vi "Initialize VDI synthesizers.vi"(11 "VDI config constants in":T3[](array[typedef])) -> (2 "Status":T1, 3 "VDI config constants out":T3[](array[typedef]))   [LabVIEW 2024, in "THz source modeule.lvlib"]
uses:
  THz source modeule.lvlib
  ctl/THz MW generator constants.ctl
  ctl/VDI status.ctl
  ctl/Synth status.ctl
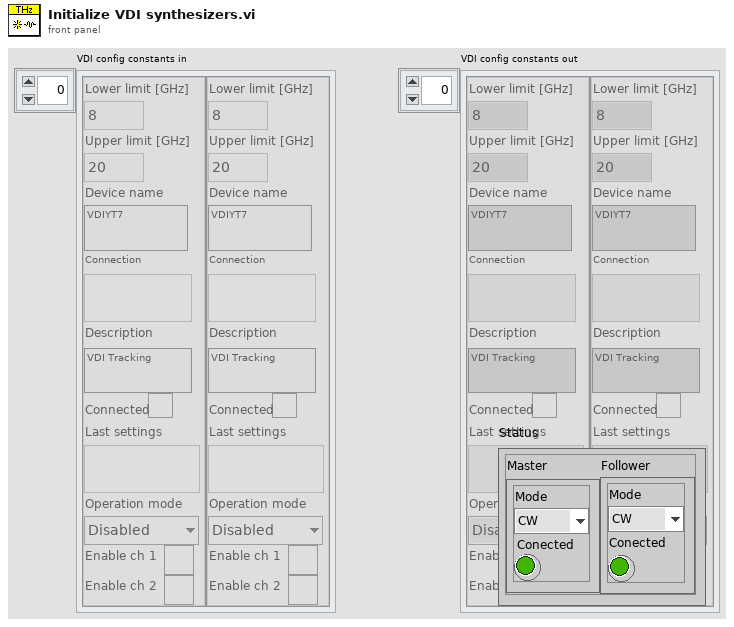
[diagram p1: front panel]
types:
  T1 = typedef "THz source modeule.lvlib/VDI status.ctl" = cluster{"Master":T2, "Follower":T2}
  T2 = typedef "THz source modeule.lvlib/Synth status.ctl" = cluster{"Mode":enum16{"CW", "Sweep"}, "Conected":bool}
  T3 = typedef "THz source modeule.lvlib/THz MW generator constants.ctl" = cluster{"Lower limit [GHz]":dbl, "Upper limit [GHz]":dbl, "Device name":string, "Connection":string, "Description":string, "Connected":bool, "Last settings":string, "Operation mode":enum16{"Disabled", "CW", "Arbitrary", "Sweep"}, "Enable ch 1":bool, "Enable ch 2":bool}
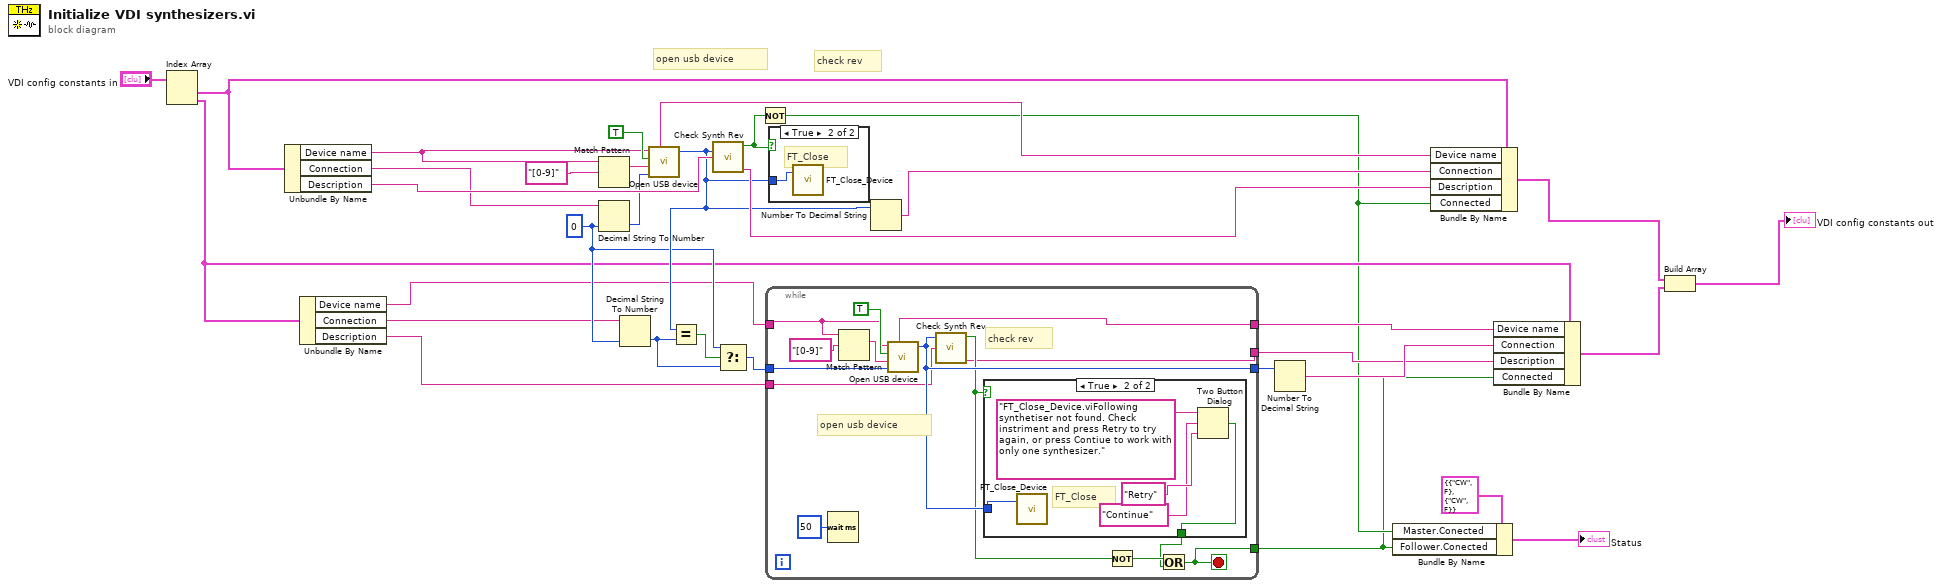
[diagram p0: block diagram]
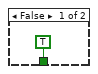
[diagram p2: hidden frame]
diagram:
  w15 = u64 0 ("default (0 I32)")
  # "check rev"
  # "open usb device"
  n1 = Index Array(array="VDI config constants in") -> (element #1=w14:T3, element #2=w7:T3)  [unwired: 2 in]
  n2 = Unbundle By Name(w14) -> ("Device name"=w6:string, "Connection"=w19:string, "Description"=w26:string)
  n3 = Unbundle By Name(w7) -> ("Device name"=w11:string, "Connection"=w12:string, "Description"=w13:string)
  n4 = Match Pattern(string=w6, regular expression="[0-9]") -> (match substring=w28:string)  [unwired: 1 in, 3 out]
  n5 = Decimal String To Number(string=w19, default (0L)=w15) -> (number=w18:u64)  [unwired: 1 in, 1 out]
  n6 = Decimal String To Number(string=w12, default (0L)=w15) -> (number=w16:u64)  [unwired: 1 in, 1 out]
  n7 = call <instrlib>:"Open USB device.vi"("SN#"=w6, "close first"=TRUE, "Prefix"=w28, "Old handle"=w18) -> ("SN# out"=w27:string, "Handle out"=w20:u64)  [unwired: 2 out]
  n8 = Equal?(x=w20, y=w16) -> (x = y?=w23:bool)
  n9 = call <instrlib>:"Check Synth Rev.vi"("Handle"=w20, "Description"=w26) -> ("Wrong Rev"=w21:bool, "Device Description"=w24:string)  [unwired: 7 in]
  n10 = Select(t=w15, s=w23, f=w16) -> (s? t:f=w22:u64)
  n11 = Not(x=w21) -> (.not. x?=w2:bool)
  n12 = while {
    tunnel: [w45] -> w1
    tunnel: w11 -> [w41]
    tunnel: [w38] -> w10
    tunnel: w13 -> [w35]
    tunnel: [w34] -> w8
    tunnel: w22 -> [w39]
    tunnel: [w37] -> w32
    stop <- w45 stop-if-true
    # "check rev"
    # "open usb device"
    n13 = Wait (ms)(milliseconds to wait=u32 50) -> ()  [unwired: 1 out]
    n14 = Match Pattern(string=w41, regular expression="[0-9]") -> (match substring=w40:string)  [unwired: 1 in, 3 out]
    n15 = call <instrlib>:"Open USB device.vi"("SN#"=w41, "close first"=TRUE, "Prefix"=w40, "Old handle"=w39) -> ("SN# out"=w38:string, "Handle out"=w37:u64)  [unwired: 2 out]
    n16 = call <instrlib>:"Check Synth Rev.vi"("Handle"=w37, "Description"=w35) -> ("Wrong Rev"=w36:bool, "Device Description"=w34:string)  [unwired: 7 in]
    n17 = case shown="True" w36 {
      tunnel: w37 -> [_ w49]
      tunnel: [TRUE ("T button?") w52] -> w44
      frame False {
      }
      frame True {
        # "FT_Close"
        n18 = call <instrlib>:"FT_Close_Device.vi"("Handle"=w49) -> ()  [unwired: 1 in, 2 out]
        n19 = Two Button Dialog(message="FT_Close_Device.viFollowing synthetiser not found. Check instriment and press Retry to try again, or press Contiue to work with only one synthesizer.", 1:"Retry" ("T button name (\"OK\")"), 2:"Continue" ("F button name (\"Cancel\")")) -> (T button?=w52:bool)
      }
    }
    n20 = Not(x=w36) -> (.not. x?=w46:bool)
    n21 = Or(x=w46, y=w44) -> (x .or. y?=w45:bool)
  }
  n22 = case shown="True" w21 {
    tunnel: w20 -> [_ w54]
    frame False {
    }
    frame True {
      # "FT_Close"
      n23 = call <instrlib>:"FT_Close_Device.vi"("Handle"=w54) -> ()  [unwired: 1 in, 2 out]
    }
  }
  n24 = Number To Decimal String(number=w20) -> (decimal integer string=w17:string)  [unwired: 1 in]
  n25 = Number To Decimal String(number=w32) -> (decimal integer string=w9:string)  [unwired: 1 in]
  n26 = Bundle By Name(cluster=T1 {"Master"={"Mode"=enum."CW", "Conected"=FALSE}, "Follower"={"Mode"=enum."CW", "Conected"=FALSE}}, "Master.Conected"=w2, "Follower.Conected"=w1) -> (→"Status":T1)
  n27 = Bundle By Name(cluster=w14, "Device name"=w27, "Connection"=w17, "Description"=w24, "Connected"=w2) -> (w4:T3)
  n28 = Bundle By Name(cluster=w7, "Device name"=w10, "Connection"=w9, "Description"=w8, "Connected"=w1) -> (w5:T3)
  n29 = Build Array(w4, w5) -> (→"VDI config constants out":T3[])
